vi "Close.vi"(8 "error in (no error)":errorcluster, 11 "reference in":refnum<class "JTAG_Base.lvclass">) -> (0 "error out":errorcluster, 3 "reference in":refnum<class "JTAG_Base.lvclass">)   [LabVIEW 2022 SP3, in "JTAG_Base.lvlib" / "JTAG_Base.lvclass"]
uses:
  JTAG_Base.lvclass
  Components/ViPER.lvlibp/ViPER.lvclass
  C:/Projects/Medulla/ViPER/Examples/Flux_Capacitor_Tester/Components/ViPER.lvlibp/ViPER.lvclass
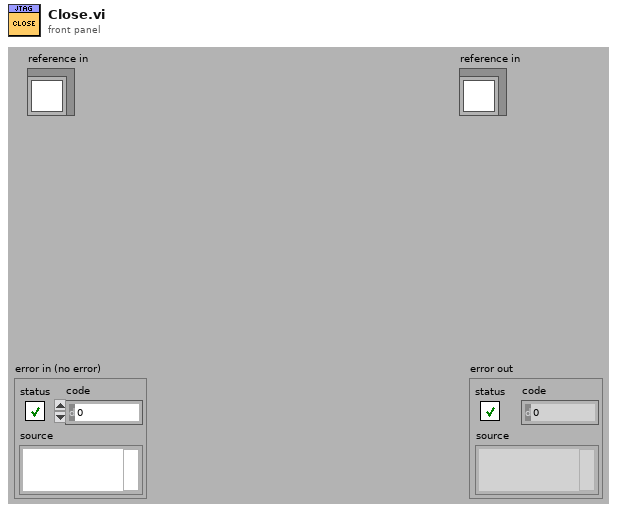
[diagram p1: front panel]
types:
  T1 = typedef "JTAG_Base.lvlib/JTAG_Base.lvclass/ObjectAttributes.ctl" = cluster{"Config":T2}
  T2 = typedef "JTAG_Base.lvlib/JTAG_Base.lvclass/Config.ctl" = cluster{"default":string}
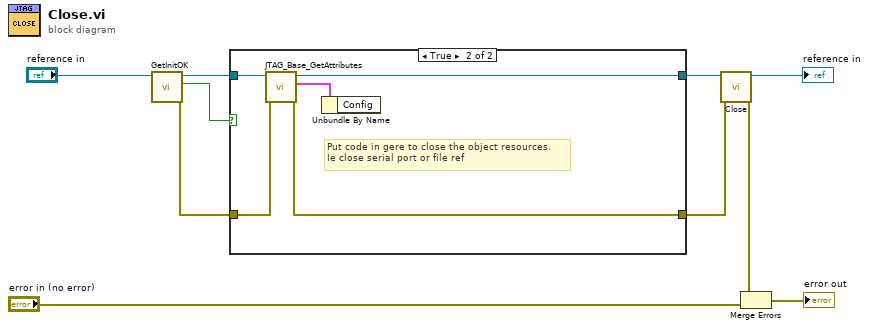
[diagram p0: block diagram]
diagram:
  n1 = call "GetInitOK.vi"("reference in"="reference in") -> ("error out"=w4:errorcluster, "init_ok"=w5:bool, "reference out"=w6:refnum<class "JTAG_Base.lvclass">)  [unwired: 8 in]
  n2 = case shown="True" w5 {
    tunnel: w4 -> [w12 w16]
    tunnel: [w12 w15] -> w7
    tunnel: w6 -> [w11 w17]
    tunnel: [w11 w13] -> w8
    frame False {
    }
    frame True {
      # "Put code in gere to close the object resources.\nIe close serial port or file ref"
      n3 = call "JTAG_Base_GetAttributes.vi"("error in (no error)"=w16, "reference in"=w17) -> ("error out"=w15:errorcluster, "Data"=w14:T1, "reference out"=w13:refnum<class "JTAG_Base.lvclass">)  [unwired: 6 in, 1 out]
      n4 = Unbundle By Name(w14) -> ()  [unwired: 1 out]
    }
  }
  n5 = call-parent "Close.vi"("error in (no error)"=w7, "reference in"=w8) -> ("error out"=w3:errorcluster, "reference out"=→"reference in":refnum<class "JTAG_Base.lvclass">)  [unwired: 8 in]
  n6 = Merge Errors(w3, "error in (no error)") -> (→"error out":errorcluster)
